vi "ATSh_SetTrigger.vi"(6 "EngineY(1)":u32=1, 7 "EngineX(0)":u32, 8 "EngineY":cluster{"Source":u32, "Slope":u32, "Level":u32}, 9 "EngineX":cluster{"Source":u32, "Slope":u32, "Level":u32}, 10 "Operation":u32, 11 "Handle":u32) -> (0 "Return":u32, 3 "Handle_Out":u32)   [LabVIEW 2015]
doc: "_____AlazarTech, Scope_____\n\nConfigure the Trigger Engine circuitry.\nHandle input.\n\nOperation:\n - Only X : 0x000\n - Only Y : 0x001\n - X or Y : 0x002\n - X and Y : 0x003\n - X xor Y : 0x004\n - X and not Y : 0x005\n - not X and Y : 0x006\n\nEngine (X and Y)\nSource:\n - Chan A : 0x000\n - Chan B : 0x001\n - External: 0x002\n - Disable : 0x003\nSlope:\n - Positive : 0x001\n - Negative: 0x002\nLevel: 0 to 255"
uses:
  ATSApi.dll
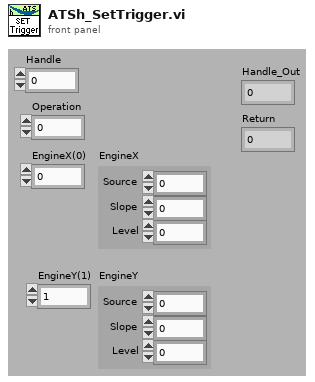
[diagram p1: front panel]
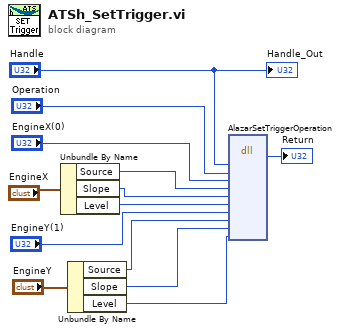
[diagram p0: block diagram]
diagram:
  n1 = Unbundle By Name("EngineX") -> ("Source"=w6:u32, "Slope"=w5:u32, "Level"=w4:u32)
  n2 = Unbundle By Name("EngineY") -> ("Source"=w7:u32, "Slope"=w8:u32, "Level"=w9:u32)
  n3 = dll-call lib="C:/IntensityOCT/trunk/ATSApi.dll" fn="AlazarSetTriggerOperation"("h"="Handle", "Operation"="Operation", "Engine1"="EngineX(0)", "Source1"=w6, "Slope1"=w5, "Level1"=w4, "Engine2"="EngineY(1)", "Source2"=w7, "Slope2"=w8, "Level2"=w9) -> (→"Return":u32)  [unwired: 13 in, 2 out]
  "Handle_Out" <- "Handle"
